vi "repair main.vi"(8 "error in":errorcluster, 10 "repair station config":T1={"Application Status"="", "Switch Output Array"=[], "Switch Value Configuration"=[], "NVH Configuration"={"NVH Station?"=FALSE, "nvh app instance path"="", "NVH_ErrorMessages sv url"="", "NVH_Inputs sv url"="", "NVH_MotionNumber sv url"="", "NVH_Outputs sv url"="", "NVH_PartNumber sv url"="", "NVH_PartNumber_Echo sv url"="", "NVH_SerialNumber sv url"="", "NVH_AmbientTempF sv url"=""}, "rs232 port map"={"PMAC"="", "PS Port"="", "LVDT Unit"="", "RS232"=""}, "ethernet address map"={"LVDT 1 Unit"="172.17.53.143", "LVDT Unit 1 port"=0}, "paths"={"Base Path"=path "", "system error log path"=path "", "Error Table Path"=path "C/Labview Code/System/Error Table", "Store errors log path"=path "C/Labview Code/System/Error Table", "data bytes log path"=path "C/Labview Code/System/Error Table", "network path"=path "C/Labview Code/System/Error Table"}, "Station Index"=0, "Store Data"={"Motion Data Array"=[], "Error Table"=[], "Sun Shade Close Force Limits"={"Overall Min"=0.0, "Overall Max"=0.0, "Avg Min"=0.0, "Avg Max"=0.0, "Truncation Start"=0.0, "Truncation End"=0.0, "Variance"=0.0, "Check Noise"=FALSE}, "Sun Shade Open Force Limits"={"Overall Min"=0.0, "Overall Max"=0.0, "Avg Min"=0.0, "Avg Max"=0.0, "Truncation Start"=0.0, "Truncation End"=0.0, "Variance"=0.0, "Check Noise"=FALSE}, "Sunshade Open Data"=[], "Sunshade Close Data"=[], "Module Info"={"Serial Number"="", "Pallet Number"="", "Sunshade Color"="", "Inalfa Part Number"="", "Customer Number"=""}, "Sunsahde Close Raw Data"=[], "Sunshade Open Raw Data"=[], "Software Version"=[], "Constant Version"=[], "Hardware Version"=[], "Inalfa Part Number ECU"=[], "LVDT Data"=[], "Communication Line 1"=[], "Communication Line 2"=[], "Anti Pinch Force"=[], "Cycle Time"="", "Anti Pinch Vent Force"=[], "iGPS LVDT Data"=[], "data bytes log"=""}, "D in map"={"Abort Test"=enum."Dev2/port2/line6", "Start Test"=enum."Dev2/port2/line6"}, "DO Task"="", "ctl refs"={"Start Test"=refnum, "Abort Test"=refnum, "Manual Control"=refnum, "Route to Repair"=refnum, "Waveform Graph"=refnum, "Motion Data"=refnum, "all station status"=refnum, "Individual Station Status"=refnum, "exit program"=refnum, "Sunshade Servo Data Open"=refnum, "Sunshade Servo Data Close"=refnum, "Red-Rabbit Mode"=refnum, "Direct Manual Ctrl"=refnum}, "misc station config"={"Station Name"="", "is AT station?"=FALSE, "is audit station?"=FALSE, "power supply type"=enum."GENser", "use alt China TP2 LVDT Logic Seq"=FALSE, "hmi operator abort timeout"=0, "dump all analog values even if pass"=FALSE, "debug log pre-filter ap stream bytes"=FALSE, "use separate lvdt x and z extend tags"=FALSE, "is print"=FALSE}, "ethernet tcp refs"={"LVDT Unit"=refnum}, "Sunshade Barcode Scan"={"Sunshade Number 2"="COM3", "Sunshade Number 1"="COM36", "Keyence tuning bank idx"=0}, "AP Test Data"={"Raw Sunshade AP Data"="", "Raw Glass AP Data"="", "PMAC Read Counter"=0.0, "Database AP Data"=[]}, "Motion Status"={"hmi operator abort start time"=0, "Current Data Index"=0, "Analog Data"=[], "Motor Position Hex"=0, "Messages Index"=0, "Last Bytes"=[], "Current Hall Position"=0, "Motion Stop Timer"=0, "Position Test"=enum."Not Tested", "Noise Test"=enum."Not Tested", "motion stop check initialized"=FALSE, "remote sense enabled"=FALSE, "Motion"=enum."Glass Teach"}, "LVDT Status"={"LVDT's stored config"=[], "lvdt precision"={"truncate instead of rounding"=FALSE, "decimal places"=0}}, "Sequence State"={"Step Description"="", "Cycle Start Time"=0, "Step Data String"="", "Pass?"=FALSE, "Seqence"=[], "Active Step"=0, "Testing?"=FALSE, "Red-Rabbit Mode"=FALSE, "route-to-repair mode"=FALSE, "NVH Status"={"Restart IRQ Counter"=0, "NVH Test Needed?"=FALSE, "NVH Test Running?"=FALSE}, "Present (s)"=0.0, "Hold Mode?"=FALSE, "Hold?"=FALSE, "Rx Invalid?"=FALSE}, "misc status"={"delay start time (ticks)"=0, "In Vehicle Mode?"=FALSE, "Diag Mode?"=FALSE, "Serial Port Configured?"=FALSE, "PS Voltage"=0.0, "Diag Serial Port"="", "Part Setup"={"Communication Type"=enum."None", "Send Messages to"=enum."Glass", "RAP Signal"=enum."High", "Motor Type"=enum."Smart Motor", "NVH Part Number"=0, "Turn Off Timer"=0, "Part Type"=""}, "Part History Number"="", "Plant Number"=0, "AP Data Type"=enum."91/61", "Real Rollo?"=FALSE}, "NVH Operator?"=FALSE, "NVH Pass?"=FALSE, "Operator Pass?"=FALSE, "Operator Action?"=FALSE, "Noise Source"=0, "USBHandle"=0, "PeakInfo"="", "PeakNumber"=0, "NVH Motion Steps"=[], "Second Check?"=FALSE, "Decibel data"=[], "Direct Control Info"={"EnableStopOnHome"=FALSE, "EnableStopOnPos"=FALSE, "TeachEvent"=FALSE, "open offset"=0, "close offset"=0, "Derect control"=FALSE, "set position"=[], "teach pass "=FALSE, "Drift offsets"=[], "Hall Positions"=[]}, "manual control(direct)"=FALSE, "LIN INFO"={"Toolkit Type"=enum."Inalfa LIN", "NAD"=36, "Inalfa LIN"={"Master Frame(3C)"="", "Slave Frame(3D)"="NIXNET_exampleLDF", "Request Schedule"="NIXNET_exampleLDF", "Response Schedule"="CEMLIN3DiagResponseSchedule\nSPA3414_ConfigurationsCMAGeely_CEMCALYPSOSDB34XX0Cfg_LIN3_190709_", "Frame Write SCU"="", "Frame Read SCU"="", "LIN Name"=""}, "ADCS LIN"={"Port"="MasterReq\nSPA3414_ConfigurationsCMAGeely_CEMCALYPSOSDB34XX0Cfg_LIN3_190709_", "HW select"=0, "XNET Cluster"="SlaveResp\nSPA3414_ConfigurationsCMAGeely_CEMCALYPSOSDB34XX0Cfg_LIN3_190709_", "ByteCmd Path"=path "C/Labview Code/System/ByteCmdConfig.txt"}, "TS LIN"={"ref info"=refnum, "LIN Channel"=0, "ByteCmd Path"=path "C/Labview Code/System/ByteCmdConfig.txt"}}, "Config Info"=variant} {"LIN INFO"."NAD" format="%.0x"; "LIN INFO"."ADCS LIN"."HW select" items=["NI-XNET", "NI-CAN"]; "LVDT Status"."LVDT's stored config"."Lower Limit" format="%.2f"; "LVDT Status"."LVDT's stored config"."Upper Limit" format="%.2f"; "Store Data"."Sun Shade Open Force Limits"."Variance" format="%.2g"; "Store Data"."Sun Shade Open Force Limits"."Truncation End" format="%.2g"; "Store Data"."Sun Shade Open Force Limits"."Truncation Start" format="%.2g"; "Store Data"."Sun Shade Open Force Limits"."Avg Max" format="%.2g"; "Store Data"."Sun Shade Open Force Limits"."Avg Min" format="%.2g"; "Store Data"."Sun Shade Open Force Limits"."Overall Max" format="%.2g"; "Store Data"."Sun Shade Open Force Limits"."Overall Min" format="%.2g"; "Store Data"."Sun Shade Close Force Limits"."Variance" format="%.2g"; "Store Data"."Sun Shade Close Force Limits"."Truncation End" format="%.2g"; "Store Data"."Sun Shade Close Force Limits"."Truncation Start" format="%.2g"; "Store Data"."Sun Shade Close Force Limits"."Avg Max" format="%.2g"; "Store Data"."Sun Shade Close Force Limits"."Avg Min" format="%.2g"; "Store Data"."Sun Shade Close Force Limits"."Overall Max" format="%.2g"; "Store Data"."Sun Shade Close Force Limits"."Overall Min" format="%.2g"; "Store Data"."Motion Data Array"."Motion Data Limits"."LIN Msg"."Msg" format="%02x"; "Store Data"."Motion Data Array"."Motion Data Limits"."LIN Msg"."ID" format="%02x"}, 11 "repair status indicator":refnum<vi>) -> (0 "error out":errorcluster)   [LabVIEW 2018]
uses:
  02.Type Def's/main state cluster.ctl
  02.Type Def's/All Switch Configuration Cluster.ctl
  02.Type Def's/All Motions.ctl
  02.Type Def's/EOL Switch Value Configuration Cluster.ctl
  02.Type Def's/EOL Switch Max Min Check Cluster.ctl
  02.Type Def's/station nvh config.ctl
  02.Type Def's/station rs232 port map.ctl
  02.Type Def's/station ethernet address map.ctl
  02.Type Def's/station paths.ctl
  02.Type Def's/EOL Save Module Test Data Control.ctl
  02.Type Def's/EOL Motion Database Table.ctl
  05.UserVI's/type defs/17x Audit Motion Data Seq Control.ctl
  05.UserVI's/type defs/17x AP Data Type.ctl
  05.UserVI's/type defs/17x Sunshade Limts Seq.ctl
  02.Type Def's/EOL Module Info Control.ctl
  02.Type Def's/station DI map.ctl
  05.UserVI's/type defs/EOL Global Digital Input Control.ctl
  02.Type Def's/control refs.ctl
  02.Type Def's/station motion data indicator.ctl
  02.Type Def's/Screen Motion Data.ctl
  02.Type Def's/Pass Fail Control.ctl
  02.Type Def's/station hmi.ctl
  02.Type Def's/lvdt name val pair.ctl
  02.Type Def's/individual station status.ctl
  02.Type Def's/misc station config.ctl
  05.UserVI's/Lambda Power/power supply types.ctl
  05.UserVI's/type defs/EOL LVDT's Check Controller.ctl
  05.UserVI's/LVDT's/lvdt precision.ctl
  02.Type Def's/sequence state.ctl
  05.UserVI's/sequence/type defs/Sequence Info.ctl
  05.UserVI's/type defs/EOL Part Setup.ctl
  02.Type Def's/All Communication Types.ctl
  05.UserVI's/type defs/Communication with Motors.ctl
  05.UserVI's/type defs/RAP Signal Control.ctl
  05.UserVI's/type defs/EOL Motor Type.ctl
  02.Type Def's/station LIN config.ctl
  03.Inalfa LIN/LIN Device.ctl
  <vilib>/CMC.AME/Inalfa ADCS/Ctl'Def/ADCS_LIN info.ctl
  C:/Program Files (x86)/National Instruments/LabVIEW 2018/vi.lib/CMC.AME/Inalfa TS LIN/TOSUN/TSMaster/bin/Interop.TSMasterAPI.dll
  Program Files (x86)/National Instruments/LabVIEW 2018/vi.lib/CMC.AME/Inalfa TS LIN/TOSUN/TSMaster/bin/Interop.TSMasterAPI.dll
  Sub'VIs/Type Def's/Config Info.ctl
  02.Type Def's/Error Data Cluster 1.0.ctl
panel:
  # "Sunroof Barcode"
  # "Pallet Number"
  # "Part Type"
  # "Application Status"
  # "Current Step"
  # "Cycle Time"
  # "Pass / Fail"
  # "Shade Close"
  # "Actual Data"
  # "Limits"
  # "Avg Current"
  # "Run Time"
  # "Speed"
  # "Noise Test"
  # "Position"
  # "Shade Open"
  # "Actual Data"
  # "Limits"
  # "Avg Current"
  # "Run Time"
  # "Speed"
  # "Noise Test"
  # "Position"
  # "Vent Close"
  # "Actual Data"
  # "Limits"
  # "Avg Current"
  # "Run Time"
  # "Speed"
  # "Noise Test"
  # "Position"
  # "Vent Open"
  # "Actual Data"
  # "Limits"
  # "Avg Current"
  # "Run Time"
  # "Speed"
  # "Noise Test"
  # "Position"
  # "Slide Close"
  # "Actual Data"
  # "Limits"
  # "Avg Current"
  # "Run Time"
  # "Speed"
  # "Noise Test"
  # "Position"
  # "Slide Open"
  # "Actual Data"
  # "Limits"
  # "Avg Current"
  # "Run Time"
  # "Speed"
  # "Noise Test"
  # "Position"
  # "Min"
  # "N"
  # "Min"
  # "Start"
  # "N"
  # "Max"
  # "N"
  # "Max"
  # "N"
  # "End"
  # "Min"
  # "N"
  # "Min"
  # "Start"
  # "N"
  # "Max"
  # "N"
  # "Max"
  # "N"
  # "End"
  # "Min"
  # "Max"
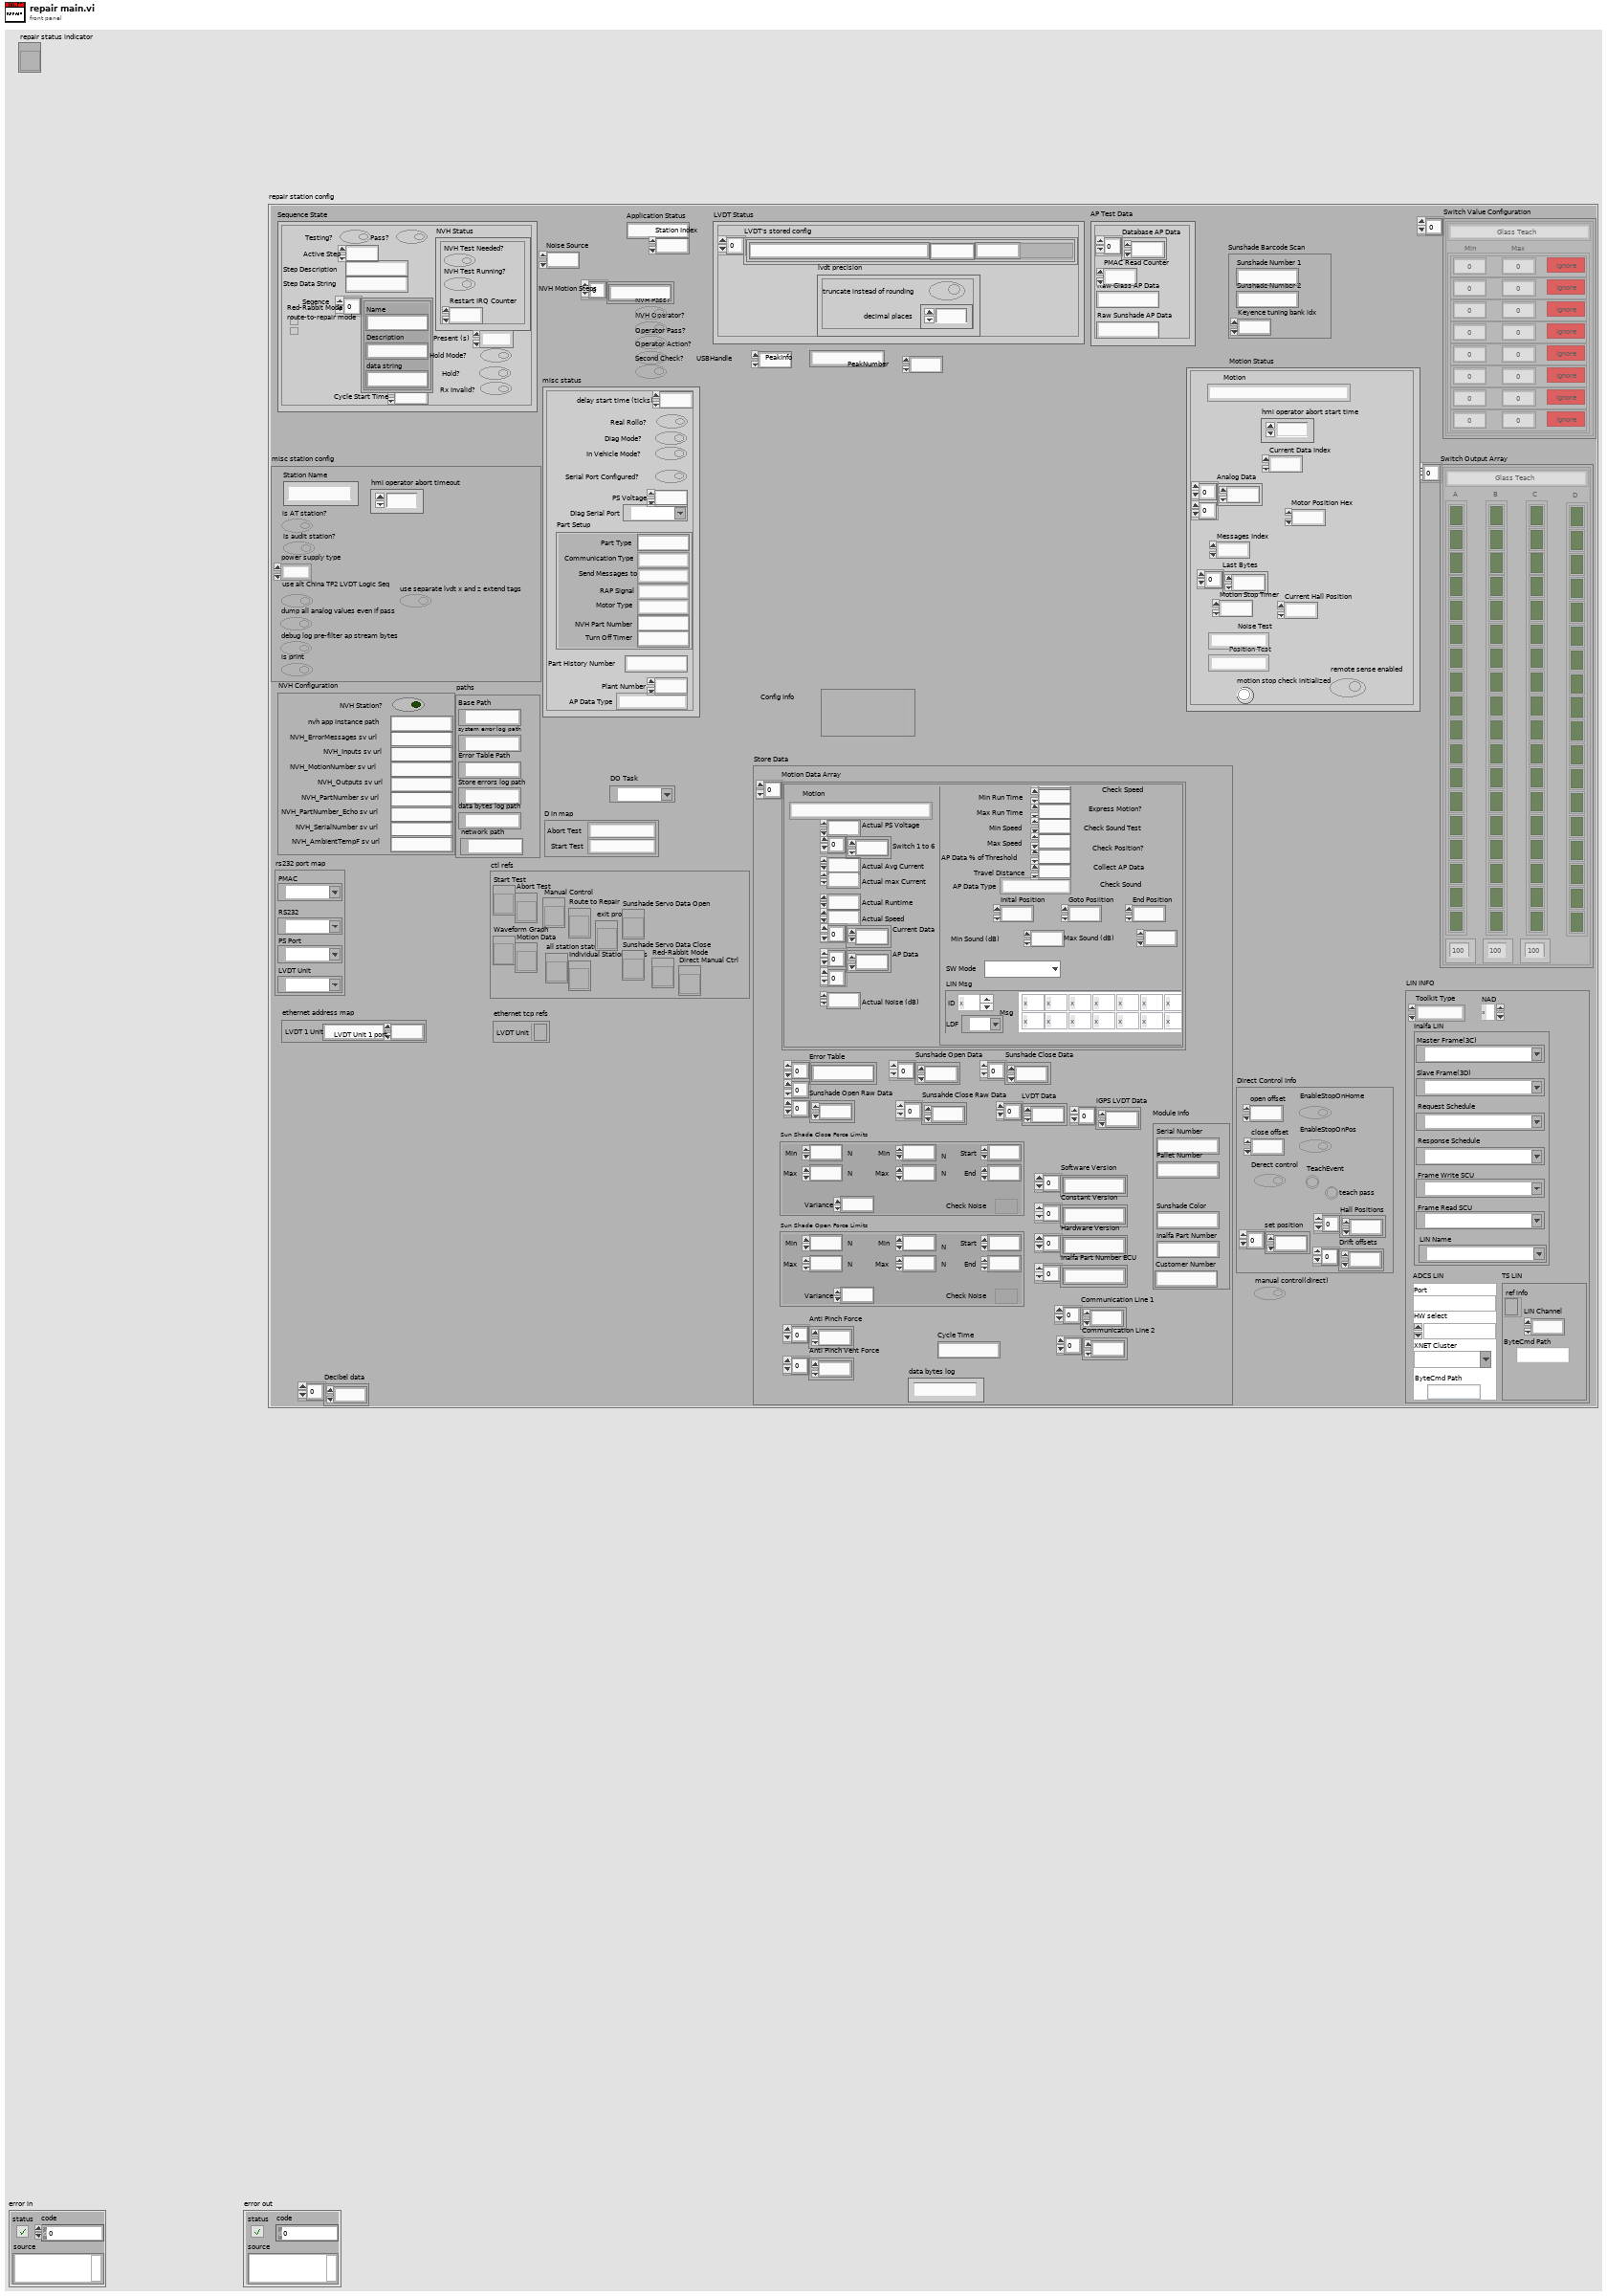
[diagram p1: front panel]
types:
  T1 = typedef "main state cluster.ctl" = cluster{"Application Status":string, "Switch Output Array":T2[], "Switch Value Configuration":T4[], "NVH Configuration":T6, "rs232 port map":T7, "ethernet address map":T8, "paths":T9, "Station Index":i32, "Store Data":T10, "D in map":T16, "DO Task":refnum<k21>, "ctl refs":T18, "misc station config":T19, "ethernet tcp refs":cluster{"LVDT Unit":refnum<k5>}, "Sunshade Barcode Scan":cluster{"Sunshade Number 2":string, "Sunshade Number 1":string, "Keyence tuning bank idx":i32}, "AP Test Data":cluster{"Raw Sunshade AP Data":string, "Raw Glass AP Data":string, "PMAC Read Counter":dbl, "Database AP Data":dbl[]}, "Motion Status":cluster{"hmi operator abort start time":u32, "Current Data Index":i32, "Analog Data":sgl[][], "Motor Position Hex":u16, "Messages Index":u16, "Last Bytes":u8[], "Current Hall Position":i16, "Motion Stop Timer":u32, "Position Test":T21, "Noise Test":T21, "motion stop check initialized":bool, "remote sense enabled":bool, "Motion":T3}, "LVDT Status":cluster{"LVDT's stored config":T22[], "lvdt precision":T23}, "Sequence State":T24, "misc status":cluster{"delay start time (ticks)":u32, "In Vehicle Mode?":bool, "Diag Mode?":bool, "Serial Port Configured?":bool, "PS Voltage":dbl, "Diag Serial Port":refnum<visa-resource-name>, "Part Setup":T26, "Part History Number":string, "Plant Number":u8, "AP Data Type":T13, "Real Rollo?":bool}, "NVH Operator?":bool, "NVH Pass?":bool, "Operator Pass?":bool, "Operator Action?":bool, "Noise Source":u32, "USBHandle":i32, "PeakInfo":string, "PeakNumber":i32, "NVH Motion Steps":string[], "Second Check?":bool, "Decibel data":dbl[], "Direct Control Info":cluster{"EnableStopOnHome":bool, "EnableStopOnPos":bool, "TeachEvent":bool, "open offset":i32, "close offset":i32, "Derect control":bool, "set position":i32[], "teach pass ":bool, "Drift offsets":i32[], "Hall Positions":i32[]}, "manual control(direct)":bool, "LIN INFO":T31, "Config Info":T34}
  T2 = typedef "All Switch Configuration Cluster.ctl" = cluster{"All Motions":T3, "A":bool[], "B":bool[], "C":bool[], "D":bool[], "A activation time (ms)":u32, "B activation time (ms)":u32, "C activation time (ms)":u32}
  T3 = typedef "All Motions.ctl" = enum16{"Glass Teach", "Glass Slide Open", "Glass Slide Close", "Glass Vent Open", "Glass Vent Close", "Sunshade Teach", "Sunshade Open", "Sunshade Close", "Idle", "Sunshade Open 2", "Sunshade Close 2", "Glass Slide Open Sunshade Open", "Glass Slide Open Sunshade Close", "Glass Slide Close Sunshade Open", "Glass Slide Close Sunshade Close", "Glass Vent Open Sunshade Open", "Glass Vent Open Sunshade Close", "Glass Vent Close Sunshade Open", "Glass Vent Close Sunshade Close", "Express Glass Slide Open", "Express Glass Slide Close", "Express Glass Vent Open", "Express Glass Vent Close", "Express Sunshade Open", "Express Sunshade Close", "Express Sunshade Open 2", "Express Sunshade Close 2", "Express Glass Slide Open Sunshade Open", "Express Glass Slide Open Sunshade Close", "Express Glass Slide Close Sunshade Open", "Express Glass Slide Close Sunshade Close", "Express Glass Vent Open Sunshade Open", "Express Glass Vent Open Sunshade Close", "Express Glass Vent Close Sunshade Open", "Express Glass Vent Close Sunshade Close", "Goto Position Glass", "Goto Position Sunshade", "Sunshade Teach 2"}
  T4 = typedef "EOL Switch Value Configuration Cluster.ctl" = cluster{"All Motions":T3, "Array":T5[]}
  T5 = typedef "EOL Switch Max Min Check Cluster.ctl" = cluster{"Min":dbl, "Max":dbl, "Check?":bool}
  T6 = typedef "station nvh config.ctl" = cluster{"NVH Station?":bool, "nvh app instance path":string, "NVH_ErrorMessages sv url":string, "NVH_Inputs sv url":string, "NVH_MotionNumber sv url":string, "NVH_Outputs sv url":string, "NVH_PartNumber sv url":string, "NVH_PartNumber_Echo sv url":string, "NVH_SerialNumber sv url":string, "NVH_AmbientTempF sv url":string}
  T7 = typedef "station rs232 port map.ctl" = cluster{"PMAC":refnum<visa-resource-name>, "PS Port":refnum<visa-resource-name>, "LVDT Unit":refnum<visa-resource-name>, "RS232":refnum<visa-resource-name>}
  T8 = typedef "station ethernet address map.ctl" = cluster{"LVDT 1 Unit":string, "LVDT Unit 1 port":u16}
  T9 = typedef "station paths.ctl" = cluster{"Base Path":path, "system error log path":path, "Error Table Path":path, "Store errors log path":path, "data bytes log path":path, "network path":path}
  T10 = typedef "EOL Save Module Test Data Control.ctl" = cluster{"Motion Data Array":T11[], "Error Table":string[][], "Sun Shade Close Force Limits":T14, "Sun Shade Open Force Limits":T14, "Sunshade Open Data":sgl[], "Sunshade Close Data":sgl[], "Module Info":T15, "Sunsahde Close Raw Data":sgl[], "Sunshade Open Raw Data":sgl[], "Software Version":string[], "Constant Version":string[], "Hardware Version":string[], "Inalfa Part Number ECU":string[], "LVDT Data":sgl[], "Communication Line 1":sgl[], "Communication Line 2":sgl[], "Anti Pinch Force":sgl[], "Cycle Time":string, "Anti Pinch Vent Force":sgl[], "iGPS LVDT Data":sgl[], "data bytes log":string}
  T11 = typedef "EOL Motion Database Table.ctl" = cluster{"Motion":T3, "Actual Avg Current":dbl, "Actual Runtime":dbl, "Actual Speed":dbl, "Current Data":sgl[], "Motion Data Limits":T12, "Switch 1 to 6":dbl[], "Actual PS Voltage":dbl, "AP Data":i16[][], "Actual max Current":dbl, "Actual Noise (dB)":dbl}
  T12 = typedef "17x Audit Motion Data Seq Control.ctl" = cluster{"Power Supply Voltage":dbl, "Min Avg Current":dbl, "Max Avg Current":dbl, "Min Run Time":dbl, "Max Run Time":dbl, "Min Speed":dbl, "Max Speed":dbl, "AP Data % of Threshold":dbl, "Travel Distance":dbl, "AP Data Type":T13, "Check Current":bool, "Check Run Time":bool, "Check Speed":bool, "Express Motion?":bool, "Check Sound Test":bool, "Check Position?":bool, "Collect AP Data":bool, "Inital Position":u16, "End Position":u16, "Goto Posiition":u16, "Max max Current":dbl, "Min max Current":dbl, "Check max Current":bool, "Check Sound":bool, "Min Sound (dB)":dbl, "Max Sound (dB)":dbl, "SW Mode":enum16{"Hard Switch", "Uncond Frame"}, "LIN Msg":cluster{"ID":u8, "Msg":u8[][], "LDF":refnum<k21>}}
  T13 = typedef "17x AP Data Type.ctl" = enum16{"91/61", "92/62", "93/63", "67", "68", "6F", "71", "91 Msg", "92 Msg", "93 Msg", "94 Msg", "HiRain 91", "HiRain 92 Speed", "HiRain 92 HS", "HiRain 92", "HiRain 93", "SnT"}
  T14 = typedef "17x Sunshade Limts Seq.ctl" = cluster{"Overall Min":dbl, "Overall Max":dbl, "Avg Min":dbl, "Avg Max":dbl, "Truncation Start":dbl, "Truncation End":dbl, "Variance":dbl, "Check Noise":bool}
  T15 = typedef "EOL Module Info Control.ctl" = cluster{"Serial Number":string, "Pallet Number":string, "Sunshade Color":string, "Inalfa Part Number":string, "Customer Number":string}
  T16 = typedef "station DI map.ctl" = cluster{"Abort Test":T17, "Start Test":T17}
  T17 = typedef "EOL Global Digital Input Control.ctl" = enum16{"Dev2/port0/line0", "Dev2/port0/line1", "Dev2/port0/line2", "Dev2/port0/line3", "Dev2/port0/line4", "Dev2/port0/line5", "Dev2/port0/line6", "Dev2/port0/line7", "Dev2/port1/line0", "Dev2/port1/line1", "Dev2/port1/line2", "Dev2/port1/line3", "Dev2/port1/line4", "Dev2/port1/line5", "Dev2/port1/line6", "Dev2/port1/line7", "Dev2/port2/line0", "Dev2/port2/line1", "Dev2/port2/line2", "Dev2/port2/line3", "Dev2/port2/line4", "Dev2/port2/line5", "Dev2/port2/line6", "Dev2/port2/line7", "Prerun Start Test", "Prerun Abort Test", "Audit Start Test", "Audit Abort Test", "Dev2/port3/line4", "Dev2/port3/line5", "Breakin Start Test", "Breakin Abort Test", "Not Implemented"}
  T18 = typedef "control refs.ctl" = cluster{"Start Test":refnum<vi>, "Abort Test":refnum<vi>, "Manual Control":refnum<vi>, "Route to Repair":refnum<vi>, "Waveform Graph":refnum<vi>, "Motion Data":refnum<vi>, "all station status":refnum<vi>, "Individual Station Status":refnum<vi>, "exit program":refnum<vi>, "Sunshade Servo Data Open":refnum<vi>, "Sunshade Servo Data Close":refnum<vi>, "Red-Rabbit Mode":refnum<vi>, "Direct Manual Ctrl":refnum<vi>}
  T19 = typedef "misc station config.ctl" = cluster{"Station Name":string, "is AT station?":bool, "is audit station?":bool, "power supply type":T20, "use alt China TP2 LVDT Logic Seq":bool, "hmi operator abort timeout":u32, "dump all analog values even if pass":bool, "debug log pre-filter ap stream bytes":bool, "use separate lvdt x and z extend tags":bool, "is print":bool}
  T20 = typedef "power supply types.ctl" = enum16{"GENser", "ZUPser", "GENeth", "Manual", "ITECH"}
  T21 = typedef "Pass Fail Control.ctl" = enum16{"Not Tested", "Pass", "Fail"}
  T22 = typedef "EOL LVDT's Check Controller.ctl" = cluster{"Upper Limit":dbl, "Lower Limit":dbl, "LVDT Name":string, "Check":bool}
  T23 = typedef "lvdt precision.ctl" = cluster{"truncate instead of rounding":bool, "decimal places":u8}
  T24 = typedef "sequence state.ctl" = cluster{"Step Description":string, "Cycle Start Time":u32, "Step Data String":string, "Pass?":bool, "Seqence":T25[], "Active Step":u8, "Testing?":bool, "Red-Rabbit Mode":bool, "route-to-repair mode":bool, "NVH Status":cluster{"Restart IRQ Counter":u8, "NVH Test Needed?":bool, "NVH Test Running?":bool}, "Present (s)":dbl, "Hold Mode?":bool, "Hold?":bool, "Rx Invalid?":bool}
  T25 = typedef "Sequence Info.ctl" = cluster{"Name":string, "Description":string, "data string":string}
  T26 = typedef "EOL Part Setup.ctl" = cluster{"Communication Type":T27, "Send Messages to":T28, "RAP Signal":T29, "Motor Type":T30, "NVH Part Number":u16, "Turn Off Timer":u16, "Part Type":string}
  T27 = typedef "All Communication Types.ctl" = enum16{"None", "CAN", "RS 232", "RS 232 LIN", "GM LIN", "SnT LIN", "K Line", "Robel CAN", "P42M-Continental", "Inalfa SCU LIN", "Spare 3"}
  T28 = typedef "Communication with Motors.ctl" = enum16{"Glass", "Rollo", "Both"}
  T29 = typedef "RAP Signal Control.ctl" = enum16{"High", "Low", "None"}
  T30 = typedef "EOL Motor Type.ctl" = enum16{"Smart Motor", "Sensor Motor"}
  T31 = typedef "station LIN config.ctl" = cluster{"Toolkit Type":enum16{"Inalfa LIN", "ADCS LIN", "TS LIN"}, "NAD":u8, "Inalfa LIN":T32, "ADCS LIN":T33, "TS LIN":cluster{"ref info":refnum<k24>, "LIN Channel":i32, "ByteCmd Path":path}}
  T32 = typedef "LIN Device.ctl" = cluster{"Master Frame(3C)":refnum<k21>, "Slave Frame(3D)":refnum<k21>, "Request Schedule":refnum<k21>, "Response Schedule":refnum<k21>, "Frame Write SCU":refnum<k21>, "Frame Read SCU":refnum<k21>, "LIN Name":refnum<k21>}
  T33 = typedef "ADCS_LIN info.ctl" = cluster{"Port":string, "HW select":u16, "XNET Cluster":string, "ByteCmd Path":path}
  T34 = typedef "Config Info.ctl" = variant
  T35 = typedef "plc comms params.ctl" = cluster{"PLC boolean read Tags":T36, "PLC bool write Tags":T39, "PLC string read Tags":T40, "PLC string write Tags":T41, "use opc":bool, "PLC/OPC Path":string}
  T36 = typedef "station plc read boolean tags.ctl" = cluster{"AT glass position":T37, "AT shade position":T37, "AT in glass wand lower pos":T37, "AT in glass wand up pos":T37, "AT in sunshad wand lower pos":T37, "AT in sunshad wand up pos":T37, "AT in wand home pos":T37, "LVDT's Extended":T37, "bolt check 1":T37, "bolt check 2":T37, "bolt check 3":T37, "bolt check 4":T37, "bolt check 5":T37, "bolt check 6":T37, "bolt check 7":T37, "bolt check 8":T37, "start":T37, "abort":T37, "LVDT's Retracted":T37, "manual barcode print":T37, "ss servo at open":T37, "ss servo at close":T37, "ss servo opening":T37, "ss servo closing":T37, "control slide at home":T37, "control slide left good":T37, "control slide left over stroke":T37, "control slide right good":T37, "control slide right over stroke":T37, "wind deflector high speed pos":T37, "wind deflector low speed pos":T37, "AT VentPMACatHome":T37, "AT VentPMACisExtend":T37, "SS Barcode Scanner Bypassed":T37, "Check Frame Barcode":T37, "Z LVDTs Extended":T37, "NVH Operator Pass":T37, "NVH Operator Fail":T37, "NVH Operator Express Glass Open":T37, "NVH Operator Express Glass Close":T37, "NVH Operator Express Rollo Open01":T37, "NVH Operator Express Rollo Close01":T37, "NVH Operator Express Rollo Open02":T37, "NVH Operator Express Rollo Close02":T37, "NVH Operator Vent Open Noise":T37, "NVH Operator Vent Close Noise":T37, "NVH Operator Sunshade Open Noise":T37, "NVH Operator Sunshade Close Noise":T37, "NVH Operator Glass Open Noise":T37, "NVH Operator Glass Close Noise":T37, "NVH Operator Finish":T37, "NVH Operator Check":T37, "windproof position":T37, "NVH Operator Express Glass vent Open":T37, "NVH Operator Express Glass Vent Close":T37, "NVH Operator Re-do":T37, "AT at vent ATS test pos":T37, "AT at vent ATS Home pos":T37, "Start Adjust LVDT":T37, "Finish Adjust LVDT":T37}
  T37 = typedef "plc path and tag.ctl" = cluster{"Tag Name":string, "Network Path":string, "use opc":bool, "DataSocket Reference":T38}
  T38 = typedef "DataSocket Reference Type.ctl" = cluster{"CWDSLib._DCWDataSocket":refnum<k7>, "CWDSLib._DCWData":refnum<k7>, "OnDataUpdated":u32, "OnStatusUpdated":u32}
  T39 = typedef "station plc write boolean tags.ctl" = cluster{"AT set glass wand lower":T37, "AT set sunshade wand lower":T37, "AT set sunshade wand up":T37, "AT set glass wand up":T37, "AT set wand home pos":T37, "Test Complete Pass":T37, "Test Complete Fail":T37, "Test Started":T37, "Retract LVDT's":T37, "Extend LVDT's":T37, "ss servo open":T37, "ss servo close":T37, "control slide start":T37, "control slide stop":T37, "AT VentPMACHome":T37, "AT VentPMACExtended":T37, "Good Frame Barcode":T37, "Bad Frame Barcode":T37, "Extend Z LVDTS":T37, "NVH SunRoof Moving":T37, "NVH SunRoof Stop":T37, "NVH Pass":T37, "NVH Fail":T37, "NVH Operator Express Glass Opened":T37, "NVH Operator Express Glass Closed":T37, "NVH Operator Express Rollo Opened01":T37, "NVH Operator Express Rollo Closed01":T37, "NVH Operator Express Rollo Opened02":T37, "NVH Operator Pass":T37, "NVH Operator Fail":T37, "NVH Operator Check":T37, "NVH Operator Vent Open Noise":T37, "NVH Operator Vent Close Noise":T37, "NVH Operator Sunshade Open Noise":T37, "NVH Operator Sunshade Close Noise":T37, "NVH Operator Glass Open Noise":T37, "NVH Operator Glass Close Noise":T37, "NVH Operator Finish":T37, "Barcode01 OK":T37, "Barcode02 OK":T37, "AT set to Vent ATS Test Pos":T37, "AT set to Vent ATS Home Pos":T37, "Move LVDT Adjust Station":T37}
  T40 = typedef "station plc read string tags.ctl" = cluster{"Serial Number":T37, "Pallet Number":T37, "Inalfa Part Number":T37, "Shade Color":T37, "Model Type":T37, "Customer Number":T37, "Part History Number":T37, "Shade 1 Barcode":T37, "Shade 2 Barcode":T37, "Manual Serial Number":T37, "Manual Inalfa Part Number":T37, "Manual Shade Color":T37, "Manual Model Type":T37, "Manual Customer Number":T37, "Manual Part History Number":T37}
  T41 = typedef "station plc write string tags.ctl" = cluster{"barcode station error":T37, "error message 0":T37, "error message 1":T37, "error message 2":T37, "error message 3":T37}
  T42 = cluster{"Base Path":path, "Module Info":T15, "Repair Station Errors":string[], "previous sn":string, "PLC Comms":T35, "repair status indicator":refnum<vi>, "Manual Control":refnum<vi>, "exit program":refnum<vi>, "Start Test":refnum<vi>, "Part Type":string}
  T43 = typedef "Error Data Cluster 1.0.ctl" = cluster{"Serial Number":string, "Error Data":string[], "Retry Counter":u8}
  T44 = typedef "repair station status.ctl" = cluster{"Loop Stopped":bool, "Error Table":string[][], "Sunroof Barcode":string, "Pallet Number":string, "Application Status":string, "Part Type":string, "Number of Times\n Module Tested":u8}
  T45 = cluster{"Serial Number":string, "Pallet Number":string, "Inalfa Part Number":string, "Part Type":string, "Shade Color":string, "Customer Number":string, "Part History Number":string, "Sunshade Barcode 2":string, "Sunshade Barcode 1":string}
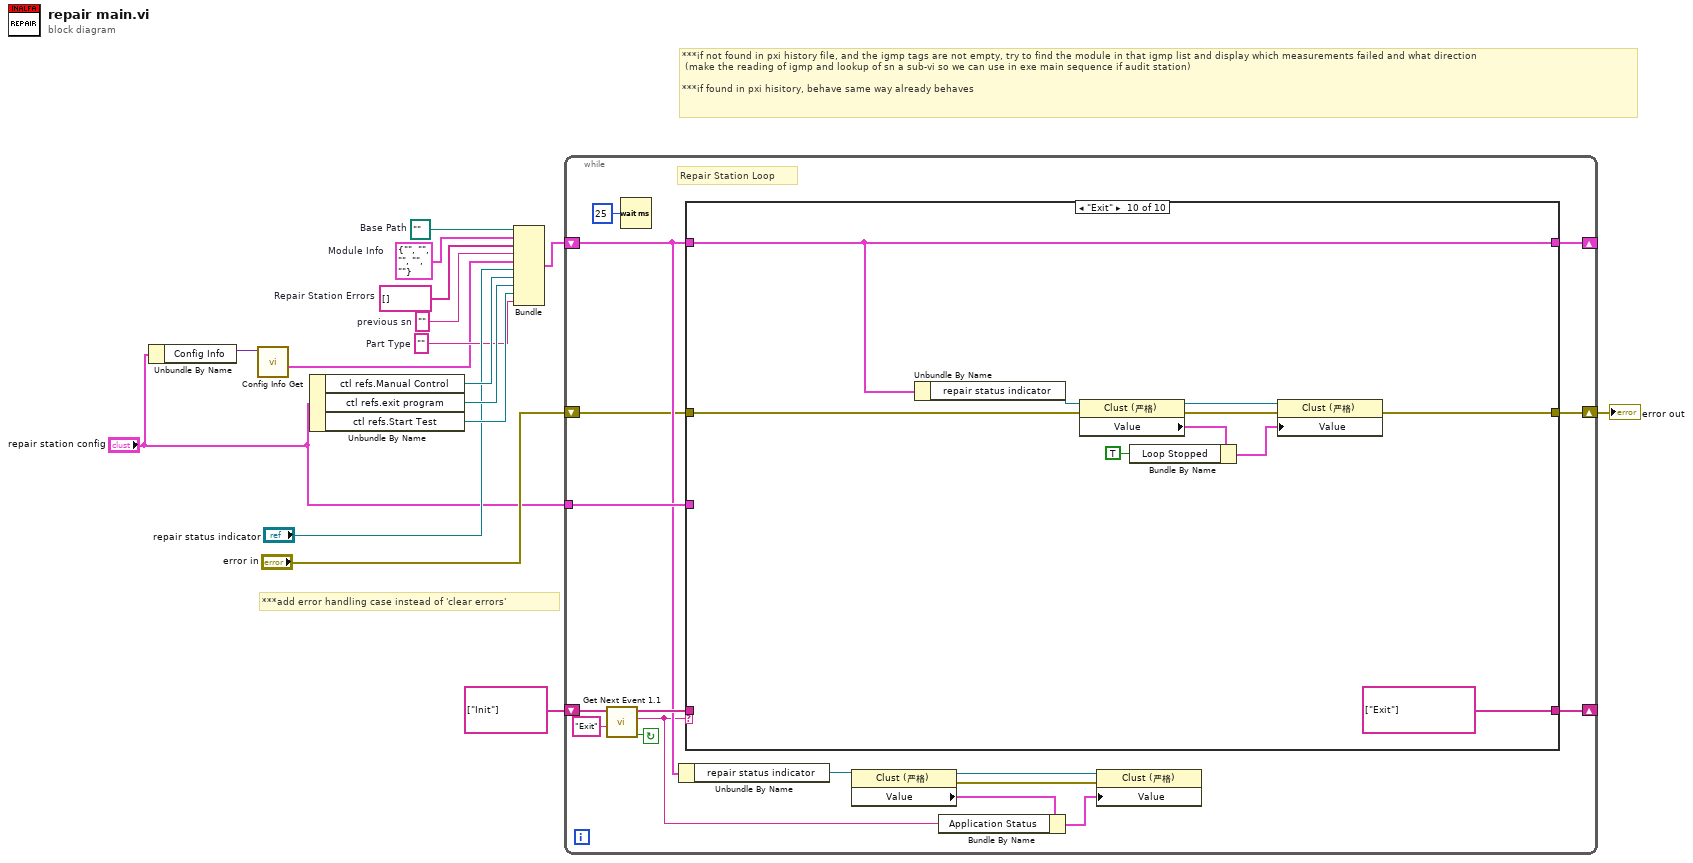
[diagram p0: block diagram]
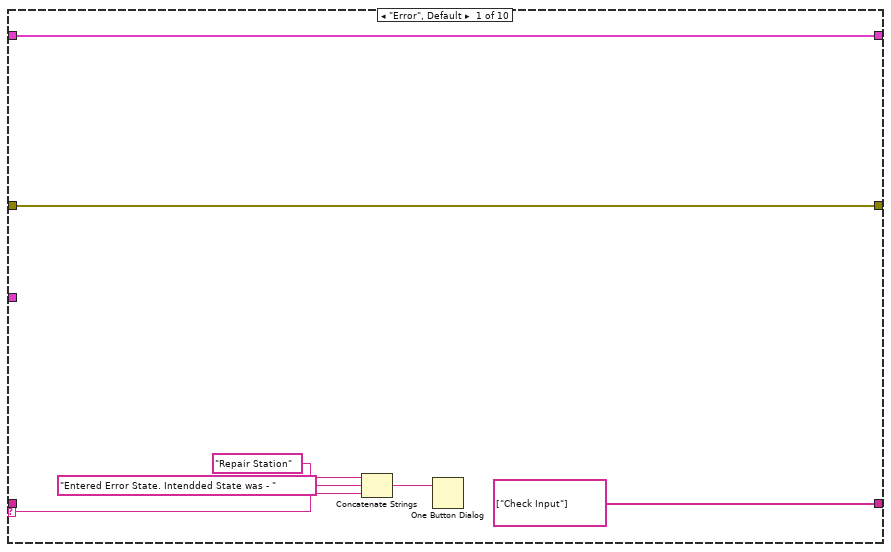
[diagram p2: hidden frame]
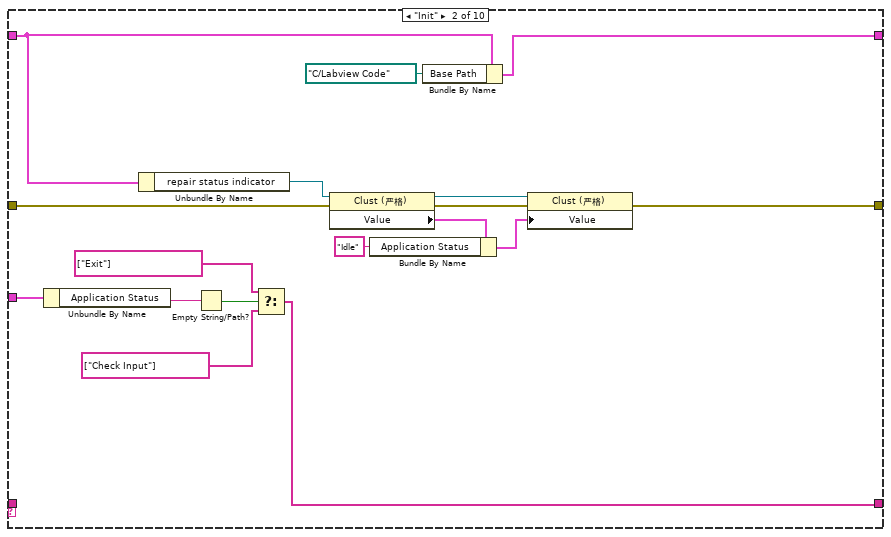
[diagram p3: hidden frame]
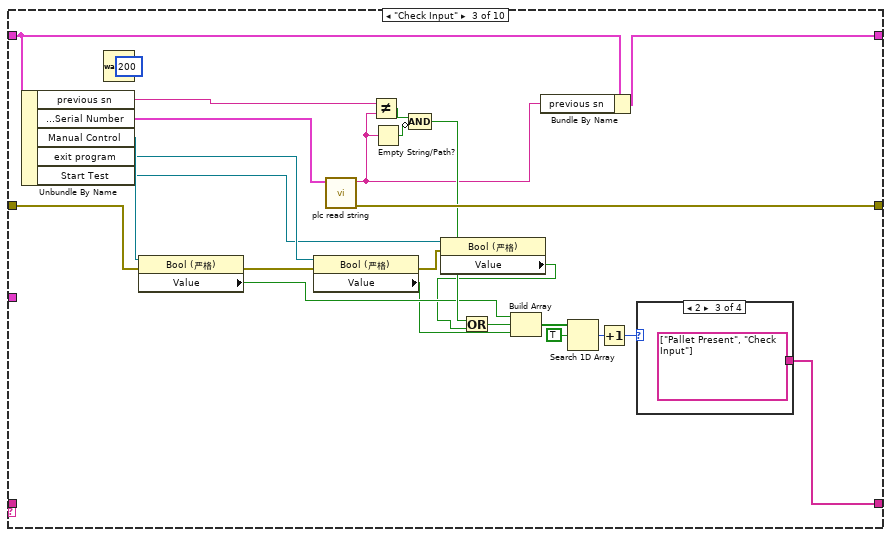
[diagram p4: hidden frame]
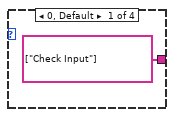
[diagram p5: hidden frame]
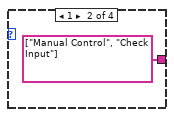
[diagram p6: hidden frame]
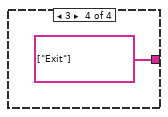
[diagram p7: hidden frame]
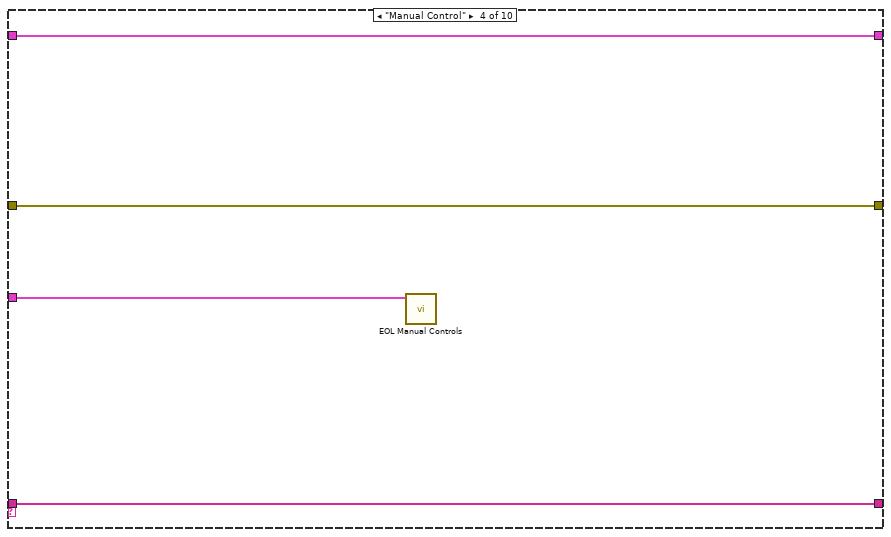
[diagram p8: hidden frame]
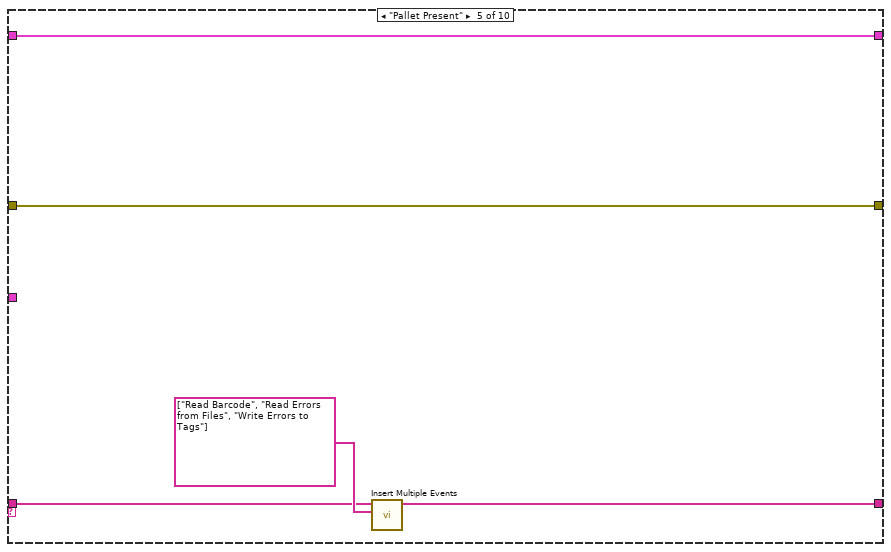
[diagram p9: hidden frame]
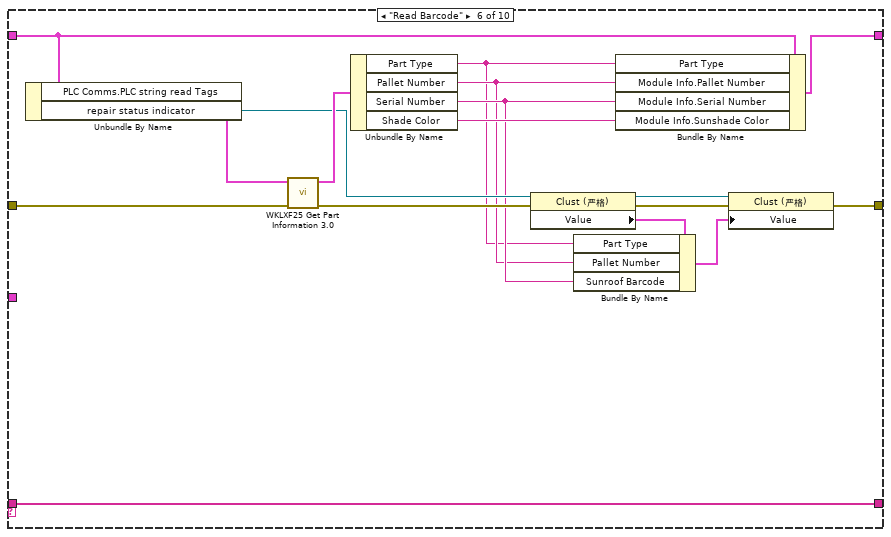
[diagram p10: hidden frame]
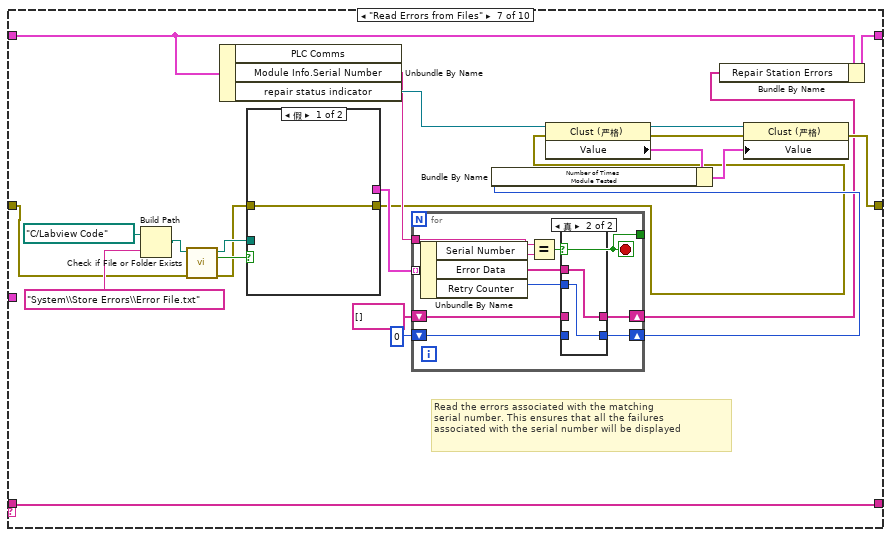
[diagram p11: hidden frame]
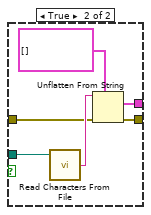
[diagram p12: hidden frame]
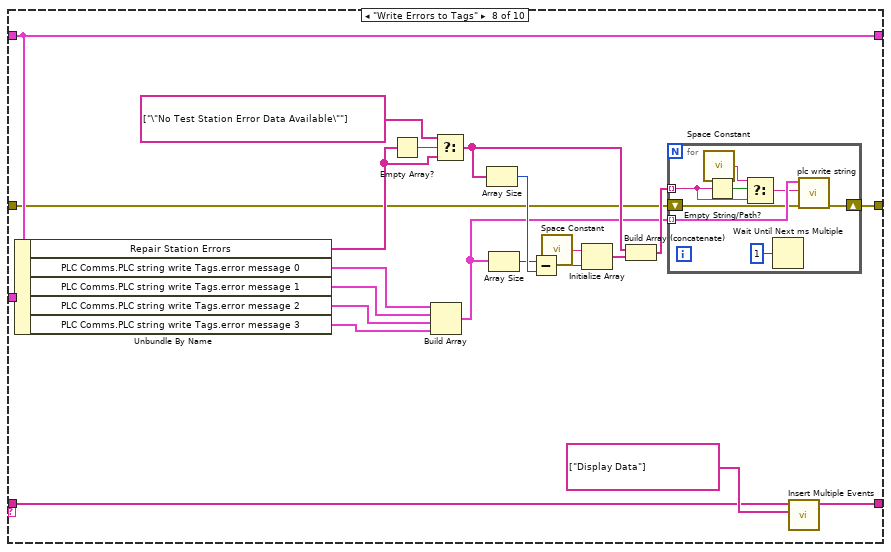
[diagram p14: hidden frame]
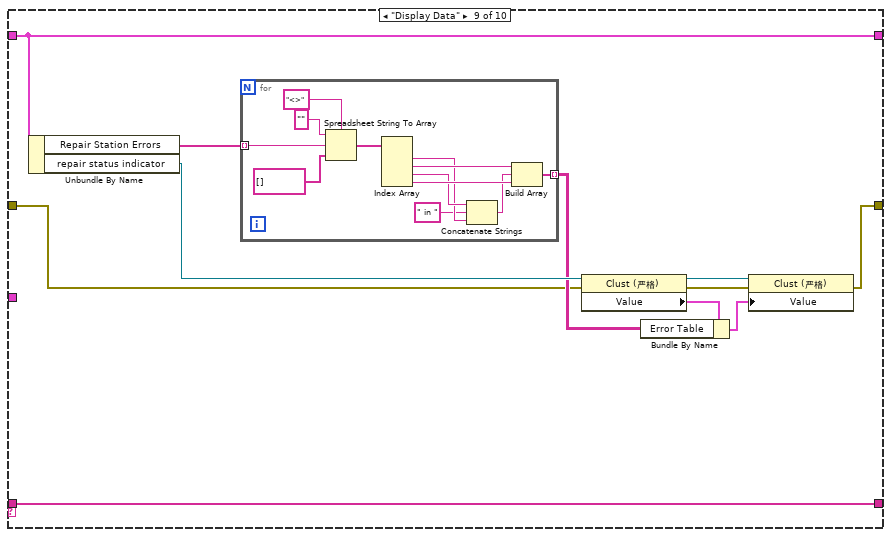
[diagram p15: hidden frame]
diagram:
  w4 = ""  # Part Type
  w12 = ""  # previous sn
  w8 = path ""  # Base Path
  w9 = T15 {"Serial Number"="", "Pallet Number"="", "Sunshade Color"="", "Inalfa Part Number"="", "Customer Number"=""}  # Module Info
  w10 = string[] []  # Repair Station Errors
  # "***if not found in pxi history file, and the igmp tags are not empty, try to find the module in that igmp list and display which measurements failed and what direction\n (make the reading of igmp and lookup of sn a sub-vi so we can use in exe main sequence if audit station)\n\n***if found in pxi hisitory, behave same way already behaves"
  # "***add error handling case instead of 'clear errors'"
  n1 = Unbundle By Name("repair station config") -> ("Config Info"=w3:T34)
  n2 = call "Config Info Get.vi"("Config Info"=w3) -> ("PLC Comms"=w1:T35)  [unwired: 7 in, 3 out]
  n3 = Unbundle By Name("repair station config") -> ("ctl refs.Manual Control"=w14:refnum<vi>, "ctl refs.exit program"=w15:refnum<vi>, "ctl refs.Start Test"=w16:refnum<vi>)
  n4 = Bundle("Base Path"=w8, "Module Info"=w9, "Repair Station Errors"=w10, "previous sn"=w12, "PLC Comms"=w1, "repair status indicator"="repair status indicator", "Manual Control"=w14, "exit program"=w15, "Start Test"=w16, "Part Type"=w4) -> (w11:T42)  [unwired: 1 in]
  n5 = while {
    shift-right: [w30] -> _
    shift-left: string[] ["Init"] ("event queue out") -> [w29]
    shift-right: [w28] -> _
    shift-left: w11 -> [w20]
    shift-right: [w26] -> w5
    shift-left: "error in" -> [w17]
    tunnel: "repair station config" -> [w25]
    stop <- w33 continue-if-true
    # "Repair Station Loop"
    n6 = call "Get Next Event 1.1.vi"("Exit Event"="Exit", "event queue in"=w29) -> ("Condition (Exit:F)"=w33:bool, "next event"=w18:string, "event queue out"=w31:string[])  [unwired: 6 in, 1 out]
    n7 = Wait (ms)(milliseconds to wait=u32 25) -> ()  [unwired: 1 out]
    n8 = Unbundle By Name(w20) -> ("repair status indicator"=w19:refnum<vi>)
    n9 = case shown="\"Exit\"" w18 {
      selector: w18 -> [w35 _ _ _ _ _ _ _ _ _]
      tunnel: w31 -> [_ _ _ w90 w92 w111 w133 w172 w196 _]
      tunnel: [string[] ["Check Input"] ("event queue out") w42 w76 w90 w93 w111 w133 w174 w196 string[] ["Exit"] ("event queue out")] -> w30
      tunnel: w20 -> [w40 w51 w75 w88 w95 w107 w135 w165 w195 w210]
      tunnel: [w40 w57 w74 w88 w95 w112 w134 w165 w195 w210] -> w28
      tunnel: [w34 w47 w70 w89 w91 w100 w122 w157 w186 w211] -> w26
      tunnel: w17 -> [w34 w48 w65 w89 w91 w106 w116 w158 w187 w212]
      tunnel: w25 -> [_ w46 _ w87 _ _ _ _ _ _]
      frame "Error", Default {
        n10 = Concatenate Strings("Repair Station" ("string"), "Entered Error State. Intendded State was - " ("string"), w35) -> (w39:string)
        n11 = One Button Dialog(message=w39) -> ()  [unwired: 1 in, 1 out]
      }
      frame "Init" {
        n12 = Unbundle By Name(w46) -> ("Application Status"=w45:string)
        n13 = Unbundle By Name(w51) -> ("repair status indicator"=w50:refnum<vi>)
        n14 = Empty String/Path?(string/path=w45) -> (empty?=w44:bool)
        n15 = Select(t=string[] ["Exit"] ("event queue out"), s=w44, f=string[] ["Check Input"] ("event queue out")) -> (s? t:f=w42:string[])
        n16 = property class="Clust (严格)"(reference=w50, error in=w48) -> (reference out=w52:refnum<vi>, error out=w53:errorcluster, "Value"=w54:T44)
        n17 = Bundle By Name(cluster=w54, "Application Status"="Idle" ("Application Status Au")) -> (w55:T44)
        n18 = Bundle By Name(cluster=w51, "Base Path"=path "C:/Labview Code") -> (w57:T42)
        n19 = property class="Clust (严格)"(reference=w52, error in=w53, "Value"=w55) -> (error out=w47:errorcluster)  [unwired: 1 out]
      }
      frame "Check Input" {
        n20 = Unbundle By Name(w75) -> ("previous sn"=w73:string, "PLC Comms.PLC string read Tags.Serial Number"=w68:T37, "Manual Control"=w64:refnum<vi>, "exit program"=w63:refnum<vi>, "Start Test"=w59:refnum<vi>)
        n21 = Wait (ms)(milliseconds to wait=u32 200) -> ()  [unwired: 1 out]
        n22 = property class="Bool (严格)"(reference=w64, error in=w65) -> (error out=w66:errorcluster, "Value"=w62:bool)  [unwired: 1 out]
        n23 = property class="Bool (严格)"(reference=w63, error in=w66) -> (error out=w60:errorcluster, "Value"=w61:bool)  [unwired: 1 out]
        n24 = call "plc read string.vi"("addr,tag"=w68) -> ("error out"=w70:errorcluster, "Data"=w67:string)  [unwired: 9 in]
        n25 = Not Equal?(x=w73, y=w67) -> (x != y?=w72:bool)
        n26 = Empty String/Path?(string/path=w67) -> (empty?=w71:bool)
        n27 = Compound Arithmetic op=AND(w72, invert w71) -> (w69:bool)
        n28 = property class="Bool (严格)"(reference=w59, error in=w60) -> ("Value"=w58:bool)  [unwired: 2 out]
        n29 = Or(x=w69, y=w58) -> (x .or. y?=w78:bool)
        n30 = Build Array(w62, w78, w61) -> (w81:bool[])
        n31 = Bundle By Name(cluster=w75, "previous sn"=w67) -> (w74:T42)
        n32 = Search 1D Array(1D array=w81, element=TRUE) -> (index of element=w79:i32)  [unwired: 1 in]
        n33 = Increment(x=w79) -> (x+1=w77:i32)
        n34 = case shown="2" w77 {
          tunnel: [string[] ["Check Input"] ("f") string[] ["Manual Control", "Check Input"] ("f") string[] ["Pallet Present", "Check Input"] ("t") string[] ["Exit"] ("t")] -> w76
          frame 0, Default {
          }
          frame 1 {
          }
          frame 2 {
          }
          frame 3 {
          }
        }
      }
      frame "Manual Control" {
        n35 = call "EOL Manual Controls.vi"("main thread cluster"=w87) -> ()  [unwired: 10 in, 1 out]
      }
      frame "Pallet Present" {
        n36 = call "Insert Multiple Events.vi"("Events to Insert"=string[] ["Read Barcode", "Read Errors from Files", "Write Errors to Tags"], "Event queue in"=w92) -> ("Event queue out"=w93:string[])  [unwired: 5 in]
      }
      frame "Read Barcode" {
        n37 = Unbundle By Name(w107) -> ("PLC Comms.PLC string read Tags"=w108:T40, "repair status indicator"=w99:refnum<vi>)
        n38 = call "WKLXF25 Get Part Information 3.0.vi"("error in"=w106, "PLC Tags"=w108) -> ("error out"=w101:errorcluster, "part info"=w110:T45)  [unwired: 7 in, 1 out]
        n39 = Unbundle By Name(w110) -> ("Part Type"=w96:string, "Pallet Number"=w97:string, "Serial Number"=w98:string, "Shade Color"=w109:string)
        n40 = property class="Clust (严格)"(reference=w99, error in=w101) -> (reference out=w102:refnum<vi>, error out=w103:errorcluster, "Value"=w104:T44)
        n41 = Bundle By Name(cluster=w104, "Part Type"=w96, "Pallet Number"=w97, "Sunroof Barcode"=w98) -> (w105:T44)
        n42 = Bundle By Name(cluster=w107, "Part Type"=w96, "Module Info.Pallet Number"=w97, "Module Info.Serial Number"=w98, "Module Info.Sunshade Color"=w109) -> (w112:T42)
        n43 = property class="Clust (严格)"(reference=w102, error in=w103, "Value"=w105) -> (error out=w100:errorcluster)  [unwired: 1 out]
      }
      frame "Read Errors from Files" {
        # "Read the errors associated with the matching \nserial number. This ensures that all the failures\nassociated with the serial number will be displayed"
        n44 = Build Path(base path=path "C:/Labview Code" ("Base Path"), name or relative path="System\\Store Errors\\Error File.txt" ("Base Path")) -> (appended path=w117:path)
        n45 = call <vilib>:"Check if File or Folder Exists.vi"("error in (no error)"=w116, "path"=w117) -> ("error out"=w113:errorcluster, "file or folder exists?"=w115:bool, "dup path"=w114:path)  [unwired: 7 in]
        n46 = Unbundle By Name(w135) -> ("Module Info.Serial Number"=w120:string, "repair status indicator"=w123:refnum<vi>)  [unwired: 1 out]
        n47 = case shown="假" w115 {
          tunnel: [_ w142] -> w131
          tunnel: [w136 w139] -> w119
          tunnel: w114 -> [_ w138]
          tunnel: w113 -> [w136 w137]
          frame False {
          }
          frame True {
            n48 = call <vilib>:"Read Characters From File.vi"("file path (dialog if empty)"=w138) -> ("character string"=w140:string)  [unwired: 5 in, 3 out]
            n49 = Unflatten From String(type=T43[] [], binary string=w140, error in (no error)=w137) -> (value=w142:T43[], error out=w139:errorcluster)  [unwired: 2 in, 1 out]
          }
        }
        n50 = for {
          tunnel: w131 -> [w152] mode=indexing
          tunnel: w120 -> [w150]
          shift-right: [w147] -> w118
          shift-left: string[] [] ("Error Data") -> [w148]
          shift-right: [w145] -> w121
          shift-left: u8 0 ("Retry Counter") -> [w144]
          tunnel: [w143] -> _
          stop <- w143 stop-if-true
          n51 = Unbundle By Name(w152) -> ("Serial Number"=w151:string, "Error Data"=w149:string[], "Retry Counter"=w146:u8)
          n52 = Equal?(x=w150, y=w151) -> (x = y?=w143:bool)
          n53 = case shown="真" w143 {
            tunnel: w149 -> [_ w156]
            tunnel: w148 -> [w154 _]
            tunnel: [w154 w156] -> w147
            tunnel: [w153 w155] -> w145
            tunnel: w146 -> [_ w155]
            tunnel: w144 -> [w153 _]
            frame False {
            }
            frame True {
            }
          }
        }
        n54 = property class="Clust (严格)"(reference=w123, error in=w119) -> (reference out=w124:refnum<vi>, error out=w125:errorcluster, "Value"=w126:T44)
        n55 = Bundle By Name(cluster=w126, "Number of Times\n Module Tested"=w121) -> (w127:T44)
        n56 = Bundle By Name(cluster=w135, "Repair Station Errors"=w118) -> (w134:T42)
        n57 = property class="Clust (严格)"(reference=w124, error in=w125, "Value"=w127) -> (error out=w122:errorcluster)  [unwired: 1 out]
      }
      frame "Write Errors to Tags" {
        n58 = Unbundle By Name(w165) -> ("Repair Station Errors"=w176:string[], "PLC Comms.PLC string write Tags.error message 0"=w163:T37, "PLC Comms.PLC string write Tags.error message 1"=w162:T37, "PLC Comms.PLC string write Tags.error message 2"=w161:T37, "PLC Comms.PLC string write Tags.error message 3"=w160:T37)
        n59 = Empty Array?(array=w176) -> (empty?=w177:bool)
        n60 = Build Array(w163, w162, w161, w160) -> (w159:T37[])
        n61 = Select(t=string[] ["\"No Test Station Error Data Available\""], s=w177, f=w176) -> (s? t:f=w169:string[])
        n62 = Array Size(array=w169) -> (size(s)=w168:i32)
        n63 = Array Size(array=w159) -> (size(s)=w164:i32)
        n64 = Subtract(x=w164, y=w168) -> (x-y=w171:i32)
        n65 = call <vilib>:"Space Constant.vi"() -> ("String"=w170:string)
        n66 = Initialize Array(w170, w171) -> (w167:string[])
        n67 = Build Array (concatenate)(w169, w167) -> (w166:string[])
        n68 = for {
          tunnel: w166 -> [w183] mode=indexing
          tunnel: w159 -> [w182] mode=indexing
          shift-right: [w179] -> w157
          shift-left: w158 -> [w180]
          n69 = call <vilib>:"Space Constant.vi"() -> ("String"=w185:string)
          n70 = Empty String/Path?(string/path=w183) -> (empty?=w184:bool)
          n71 = Select(t=w185, s=w184, f=w183) -> (s? t:f=w181:string)
          n72 = Wait Until Next ms Multiple(millisecond multiple=u32 1) -> ()  [unwired: 1 out]
          n73 = call "plc write string.vi"("error in"=w180, "value"=w181, "addr,tag"=w182) -> ("error out"=w179:errorcluster)  [unwired: 8 in]
        }
        n74 = call "Insert Multiple Events.vi"("Events to Insert"=string[] ["Display Data"], "Event queue in"=w172) -> ("Event queue out"=w174:string[])  [unwired: 5 in]
      }
      frame "Display Data" {
        n75 = Unbundle By Name(w195) -> ("Repair Station Errors"=w194:string[], "repair status indicator"=w189:refnum<vi>)
        n76 = for {
          tunnel: w194 -> [w206] mode=indexing
          tunnel: [w199] -> w188 mode=indexing
          n77 = Spreadsheet String To Array(delimiter (Tab)="<>", format string="", spreadsheet string=w206, array type (2D Dbl)=string[] [] ("Error Data")) -> (array=w204:string[])
          n78 = Index Array(array=w204) -> (element #1=w198:string, element #2=w203:string, element #3=w201:string, element #4=w202:string)  [unwired: 4 in]
          n79 = Concatenate Strings(w201, " in " ("string"), w198) -> (w200:string)
          n80 = Build Array(w203, w200, w202) -> (w199:string[])
        }
        n81 = property class="Clust (严格)"(reference=w189, error in=w187) -> (reference out=w190:refnum<vi>, error out=w191:errorcluster, "Value"=w192:T44)
        n82 = Bundle By Name(cluster=w192, "Error Table"=w188) -> (w193:T44)
        n83 = property class="Clust (严格)"(reference=w190, error in=w191, "Value"=w193) -> (error out=w186:errorcluster)  [unwired: 1 out]
      }
      frame "Exit" {
        n84 = Unbundle By Name(w210) -> ("repair status indicator"=w209:refnum<vi>)
        n85 = property class="Clust (严格)"(reference=w209, error in=w212) -> (reference out=w214:refnum<vi>, error out=w215:errorcluster, "Value"=w216:T44)
        n86 = Bundle By Name(cluster=w216, "Loop Stopped"=TRUE ("Boolean")) -> (w217:T44)
        n87 = property class="Clust (严格)"(reference=w214, error in=w215, "Value"=w217) -> (error out=w211:errorcluster)  [unwired: 1 out]
      }
    }
    n88 = property class="Clust (严格)"(reference=w19) -> (reference out=w21:refnum<vi>, error out=w22:errorcluster, "Value"=w23:T44)  [unwired: 1 in]
    n89 = Bundle By Name(cluster=w23, "Application Status"=w18) -> (w24:T44)
    n90 = property class="Clust (严格)"(reference=w21, error in=w22, "Value"=w24) -> ()  [unwired: 2 out]
  }
  "error out" <- w5
